vi "printErrorList.vi"(8 "error in (no error)":errorcluster, 9 "Errors":T1, 10 "flavor":string, 11 "TestTestResult in":refnum<class "_TextTestResult.lvclass">) -> (0 "error out":errorcluster, 3 "TestTestResult out":refnum<class "_TextTestResult.lvclass">)   [LabVIEW 2013, in "_TextTestResult.lvclass"]
uses:
  _TextTestResult.lvclass
  TestResult/private/errors.ctl
  TestResult/private/error.ctl
  _TextTestResult.lvclass/_TextTestResult.ctl
  TestResult/TestResult.lvclass
panel:
  # "JKI VI Tester for LabVIEW\nhttp://jkisoft.com/vi-tester\nCopyright (C) 2007-2009, JKI <info@jkisoft.com>\nALL RIGHTS RESERVED"
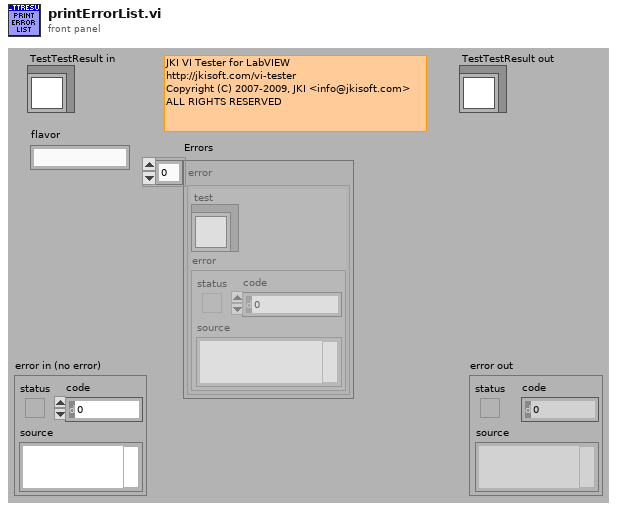
[diagram p1: front panel]
types:
  T1 = typedef "TestResult.lvclass/errors.ctl" = T2[]
  T2 = typedef "TestResult.lvclass/error.ctl" = cluster{"test":refnum<class>, "error":errorcluster}
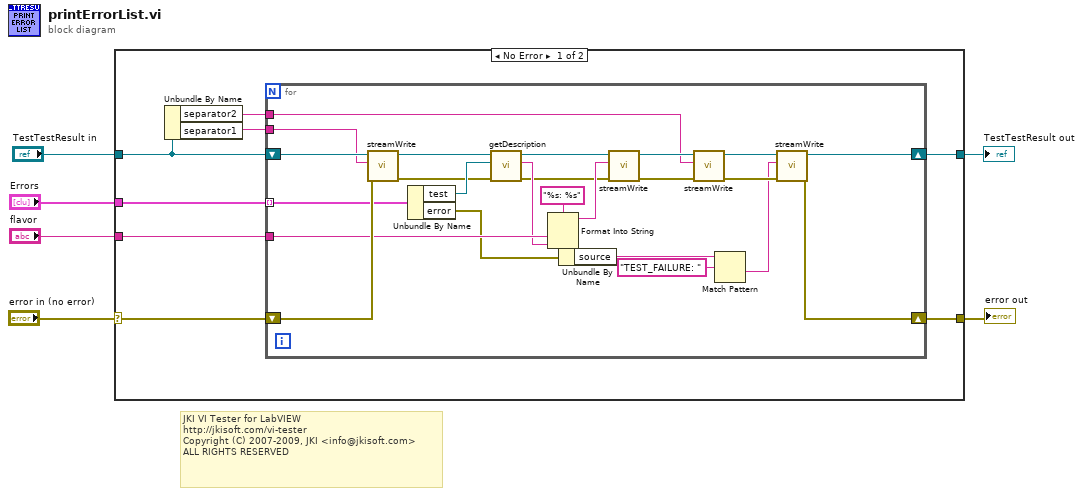
[diagram p0: block diagram]
diagram:
  # "JKI VI Tester for LabVIEW\nhttp://jkisoft.com/vi-tester\nCopyright (C) 2007-2009, JKI <info@jkisoft.com>\nALL RIGHTS RESERVED"
  n1 = case shown="No Error" "error in (no error)" {
    selector: "error in (no error)" -> [w11 w40]
    tunnel: [w10 w40] -> w5
    tunnel: [w12 w39] -> w3
    tunnel: "TestTestResult in" -> [w9 w39]
    tunnel: "Errors" -> [w14 _]
    tunnel: "flavor" -> [w13 _]
    frame No Error {
      n2 = Unbundle By Name(w9) -> ("separator2"=w8:string, "separator1"=w7:string)
      n3 = for {
        tunnel: w14 -> [w35] mode=indexing
        shift-right: [w26] -> w10
        shift-left: w11 -> [w38]
        shift-right: [w24] -> w12
        shift-left: w9 -> [w16]
        tunnel: w13 -> [w36]
        tunnel: w8 -> [w17]
        tunnel: w7 -> [w15]
        n4 = call "streamWrite.vi"("error in (no error)"=w38, "String"=w15, "TestTestResult in"=w16) -> ("error out"=w21:errorcluster, "TestTestResult out"=w31:refnum<class "_TextTestResult.lvclass">)  [unwired: 7 in]
        n5 = Unbundle By Name(w35) -> ("test"=w34:refnum<class>, "error"=w28:errorcluster)
        n6 = call-dynamic "getDescription.vi"("error in (no error)"=w21, "test"=w34, "TestTestResult in"=w31) -> ("error out"=w22:errorcluster, "description"=w33:string, "TestTestResult in"=w30:refnum<class "_TextTestResult.lvclass">)  [unwired: 6 in]
        n7 = Format Into String(format string="%s: %s", w36, w33) -> (resulting string=w32:string)  [unwired: 2 in, 1 out]
        n8 = Unbundle By Name(w28) -> ("source"=w19:string)
        n9 = call "streamWrite.vi"("error in (no error)"=w22, "String"=w32, "TestTestResult in"=w30) -> ("error out"=w23:errorcluster, "TestTestResult out"=w29:refnum<class "_TextTestResult.lvclass">)  [unwired: 7 in]
        n10 = call "streamWrite.vi"("error in (no error)"=w23, "String"=w17, "TestTestResult in"=w29) -> ("error out"=w27:errorcluster, "TestTestResult out"=w25:refnum<class "_TextTestResult.lvclass">)  [unwired: 7 in]
        n11 = Match Pattern(string=w19, regular expression="TEST_FAILURE: ") -> (after substring=w18:string)  [unwired: 1 in, 3 out]
        n12 = call "streamWrite.vi"("error in (no error)"=w27, "String"=w18, "TestTestResult in"=w25) -> ("error out"=w26:errorcluster, "TestTestResult out"=w24:refnum<class "_TextTestResult.lvclass">)  [unwired: 7 in]
      }
    }
    frame Error {
    }
  }
  "error out" <- w5
  "TestTestResult out" <- w3
